vi "Query discriminator level (scan).vi"(8 "error in (no error)":errorcluster, 10 "i (0)":T1, 11 "VISA resource name":refnum<visa-resource-name>) -> (0 "error out":errorcluster, 2 "output":dbl, 3 "VISA resource name out":refnum<visa-resource-name>)   [LabVIEW 2015, in "SR400.lvlib"]
doc: "DZ i\nThe DZ command returns the level of\ndiscriminator i during a scan. i = 0,1, or 2\ndesignates discriminator A,B, or T and is required.\nIf discriminator i is in the SCAN mode, its current\nlevel during a scan is read. If the counters are in\nreset or the discriminator is in the FIXED mode,\nthe DZ command returns the starting value for the\nlevel (same as DL command). The DZ command\nis a read only command."
uses:
  SR400.lvlib
  Typedefs/Counter.ctl
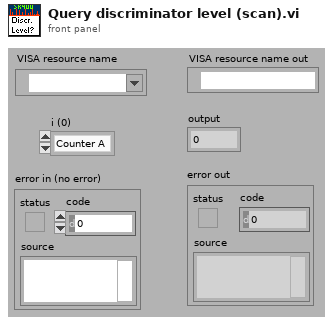
[diagram p1: front panel]
types:
  T1 = typedef "SR400.lvlib/Counter.ctl" = enum16{"Counter A", "Counter B", "Counter T"}
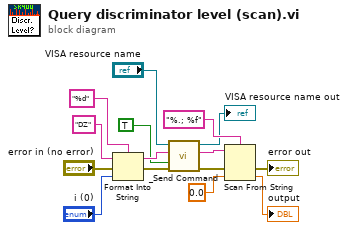
[diagram p0: block diagram]
diagram:
  n1 = Format Into String(format string="%d", initial string="DZ" ("command"), error in="error in (no error)", "i (0)") -> (resulting string=w6:string, error out=w5:errorcluster)
  n2 = call "_Send Command.vi"("error in (no error)"=w5, "Query? (F)"=TRUE, "Command"=w6, "VISA resource name"="VISA resource name") -> ("error out"=w2:errorcluster, "Response"=w3:string, "VISA resource name out"=→"VISA resource name out":refnum<visa-resource-name>)  [unwired: 5 out]
  n3 = Scan From String(format string="%.; %f", input string=w3, error in=w2, default 1=0.0 ("default value 1")) -> (error out=→"error out":errorcluster, output 1=→"output":dbl)  [unwired: 1 in, 2 out]
